vi "Get Static Member VIs.vi"(8 "error in (no error)":errorcluster, 10 "Test Class Path":path) -> (0 "error out":errorcluster, 1 "VI Names":set{string}(c389), 2 "Array":path[](array[path]))   [LabVIEW 2020, in "Responsive Mock Class Generator Test.lvclass"]
uses:
  Responsive Mock Class Generator Test.lvclass
  Responsive Mock Class Generator Test.lvclass/Responsive Mock Class Generator Test.ctl
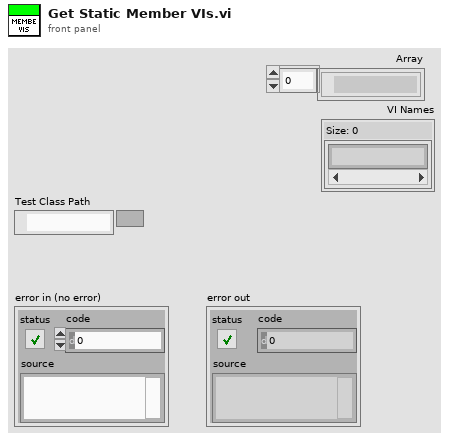
[diagram p1: front panel]
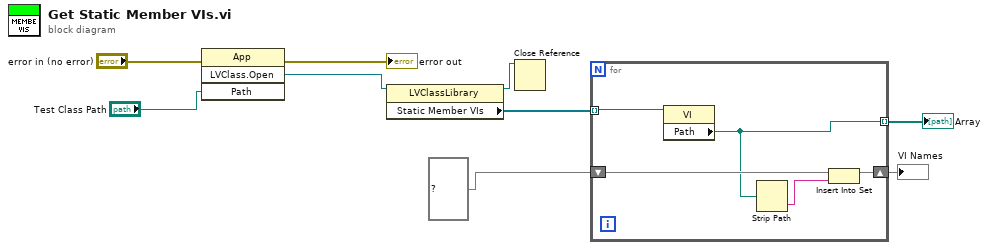
[diagram p0: block diagram]
diagram:
  n1 = invoke class="App" method="LVClass.Open"(error in="error in (no error)", "Path"="Test Class Path") -> (error out=→"error out":errorcluster, "LVClass.Open"=w6:refnum<vi>)  [unwired: 2 in, 2 out]
  n2 = property class="LVClassLibrary"(reference=w6) -> (reference out=w5:refnum<vi>, "Static Member VIs"=w4:refnum<vi>[])  [unwired: 1 in, 1 out]
  n3 = Close Reference(reference=w5) -> ()  [unwired: 1 in, 1 out]
  n4 = for {
    tunnel: w4 -> [w14] mode=indexing
    tunnel: [w11] -> w3 mode=indexing
    shift-right: [w12] -> w1
    shift-left: set{string} {} ("set") -> [w13]
    n5 = property class="VI"(reference=w14) -> ("Path"=w11:path)  [unwired: 1 in, 2 out]
    n6 = Strip Path(path=w11) -> (name=w10:string)  [unwired: 1 out]
    n7 = Insert Into Set(10:w10, 11:w13) -> (3:w12:set{string})  [unwired: 1 out]
  }
  "Array" <- w3
  "VI Names" <- w1
